vi "Unflatten.vi"(8 "error in (no error)":errorcluster, 9 "timeout in":bool, 10 "Data In":refnum<data-value>[](array[refnum]), 11 "CIFFifoCAN in":refnum<class "CIF_NIChn_Fifo_Power_DVR.lvclass">) -> (0 "error out":errorcluster, 2 "Data Out":refnum<data-value>[](array[refnum]), 3 "CIFFifoCAN out":refnum<class "CIF_NIChn_Fifo_Power_DVR.lvclass">, 4 "Header":T1)   [LabVIEW 2021, in "CIF_NIChn_Fifo_Power_DVR.lvclass"]
uses:
  CIF_NIChn_Fifo_Power_DVR.lvclass
  ChannelCommon/CIFFIFO/CIFfifo.lvclass
  ChannelCommon/typedef/FIFO Header.ctl
  ChannelCommon/ChannelCommon.lvlib
  ChannelCommon/typedef/Datatype Waveform.ctl
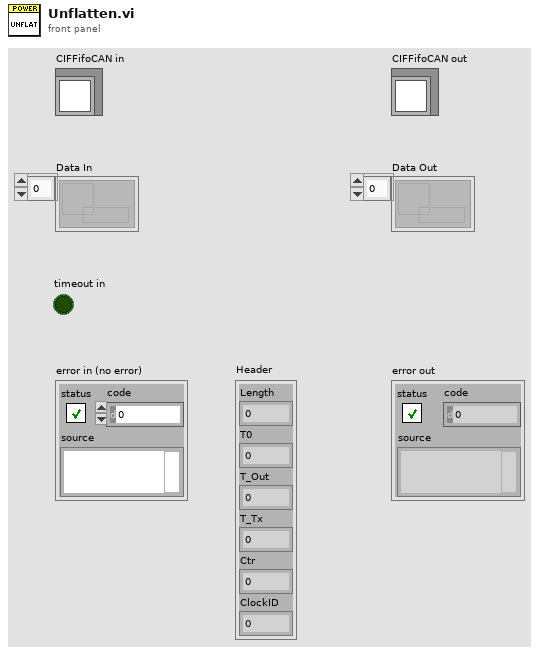
[diagram p1: front panel]
types:
  T1 = typedef "ChannelCommon.lvlib/FIFO Header.ctl" = cluster{"Length":u64, "T0":i64, "T_Out":i64, "T_Tx":i64, "Ctr":u64, "ClockID":u8}
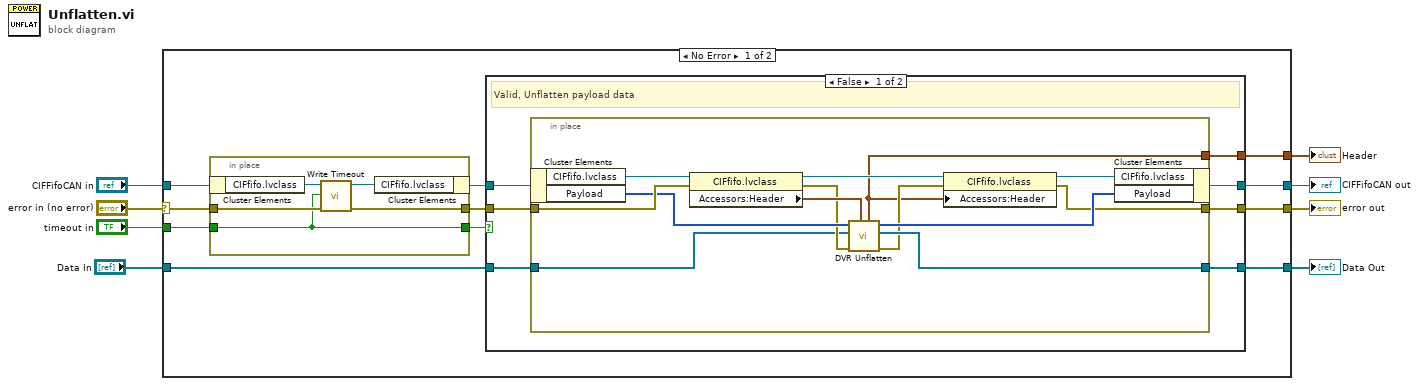
[diagram p0: block diagram]
diagram:
  n1 = case shown="No Error" "error in (no error)" {
    selector: "error in (no error)" -> [w18 w49]
    tunnel: [w11 w49] -> w7
    tunnel: [w12 w48] -> w5
    tunnel: "CIFFifoCAN in" -> [w19 w48]
    tunnel: "timeout in" -> [w17 _]
    tunnel: [w14 _] -> w2
    tunnel: [w13 _] -> w3
    tunnel: "Data In" -> [w9 _]
    frame No Error {
      n2 = in-place {
        in-place-border: w18 -> [w45]
        in-place-border: [w44] -> w16
        in-place-border: w17 -> [w43]
        in-place-border: [w43] -> w10
        n3 = in-place-cluster #1(w19) -> ("CIFfifo.lvclass"=w47:refnum<class "CIFfifo.lvclass">)
        n4 = call "Write Timeout.vi"("error in (no error)"=w45, "Timeout"=w43, "CIFFIFO in"=w47) -> ("error out"=w44:errorcluster, "CIFFIFO out"=w46:refnum<class "CIFfifo.lvclass">)  [unwired: 7 in]
        n5 = in-place-cluster #1("CIFfifo.lvclass"=w46) -> (w15:refnum<class "CIF_NIChn_Fifo_Power_DVR.lvclass">)
      }
      n6 = case shown="False" w10 {
        tunnel: w16 -> [w26 w41]
        tunnel: w15 -> [w25 w42]
        tunnel: [w24 w40] -> w14
        tunnel: [w23 _] -> w13
        tunnel: [w22 w42] -> w12
        tunnel: [w21 w41] -> w11
        tunnel: w9 -> [w20 w40]
        frame False {
          # "Valid, Unflatten payload data"
          n7 = in-place {
            in-place-border: w26 -> [w39]
            in-place-border: [w34] -> w24
            in-place-border: [w28] -> w23
            in-place-border: [w29] -> w21
            in-place-border: w20 -> [w27]
            n8 = in-place-cluster #2(w25) -> ("CIFfifo.lvclass"=w37:refnum<class "CIFfifo.lvclass">, "Payload"=w33:u8[])
            n9 = property class="CIFfifo.lvclass"(reference=w37, error in=w39) -> (reference out=w38:refnum<class "CIFfifo.lvclass">, error out=w31:errorcluster, "Accessors:Header"=w32:T1)
            n10 = call "DVR Unflatten.vi"("Header in"=w32, "error in (no error)"=w31, "DVRs In"=w27, "Flatten Data in"=w33) -> ("error out"=w30:errorcluster, "DVRs Out"=w34:refnum<data-value>[], "Flatten Data out"=w35:u8[], "Header out"=w28:T1)  [unwired: 4 in]
            n11 = property class="CIFfifo.lvclass"(reference=w38, error in=w30, "Accessors:Header"=w28) -> (reference out=w36:refnum<class "CIFfifo.lvclass">, error out=w29:errorcluster)
            n12 = in-place-cluster #2("CIFfifo.lvclass"=w36, "Payload"=w35) -> (w22:refnum<class "CIF_NIChn_Fifo_Power_DVR.lvclass">)
          }
        }
        frame True {
          # "Timeout"
        }
      }
    }
    frame Error {
    }
  }
  "error out" <- w7
  "CIFFifoCAN out" <- w5
  "Header" <- w3
  "Data Out" <- w2
